vi "TDMS Record.vi"(9 "Data":dbl[][](array[numeric]), 10 "Input TDMS File Cluster":T1, 11 "In Use Cluster":T2) -> (3 "Output TDMS File Cluster":T1)   [LabVIEW 2014]
panel:
  # "TDMS Record VI"
  # "Inputs"
  # "Outputs"
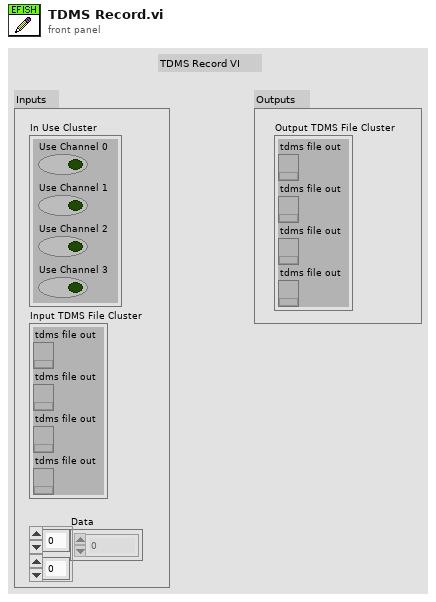
[diagram p1: front panel]
types:
  T1 = cluster{"tdms file out":refnum<k34>, "tdms file out":refnum<k34>, "tdms file out":refnum<k34>, "tdms file out":refnum<k34>}
  T2 = cluster{"Use Channel 0":bool, "Use Channel 1":bool, "Use Channel 2":bool, "Use Channel 3":bool}
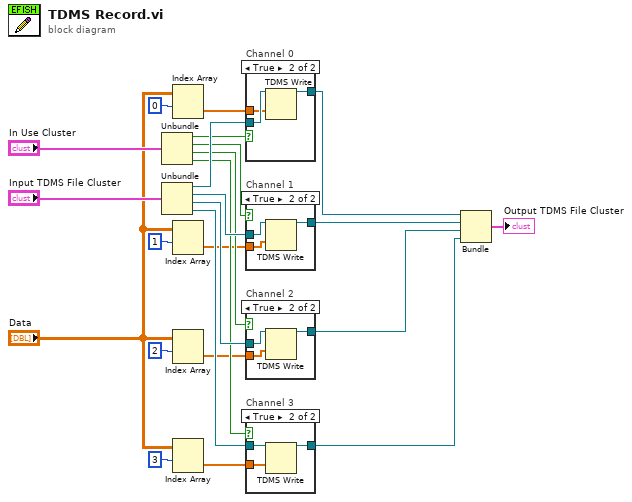
[diagram p0: block diagram]
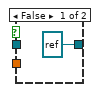
[diagram p2: hidden frame]
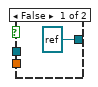
[diagram p3: hidden frame]
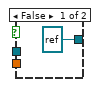
[diagram p4: hidden frame]
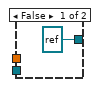
[diagram p5: hidden frame]
diagram:
  n1 = Unbundle("In Use Cluster") -> ("Use Channel 0"=w22:bool, "Use Channel 1"=w17:bool, "Use Channel 2"=w16:bool, "Use Channel 3"=w15:bool)
  n2 = Unbundle("Input TDMS File Cluster") -> ("tdms file out"=w24:refnum<k34>, "tdms file out"=w20:refnum<k34>, "tdms file out"=w19:refnum<k34>, "tdms file out"=w18:refnum<k34>)
  n3 = Index Array(array="Data", index (row)=0) -> (element=w13:dbl[])  [unwired: 1 in]
  n4 = Index Array(array="Data", index (row)=1) -> (element=w11:dbl[])  [unwired: 1 in]
  n5 = Index Array(array="Data", index (row)=2) -> (element=w9:dbl[])  [unwired: 1 in]
  n6 = Index Array(array="Data", index (row)=3) -> (element=w6:dbl[])  [unwired: 1 in]
  n7 = case "Channel 0" shown="True" w22 {
    tunnel: w24 -> [_ w28]
    tunnel: [refnum<k34> refnum ("tdms file out") w27] -> w5
    tunnel: w13 -> [_ w26]
    frame False {
    }
    frame True {
      n8 = TDMS Write(0:w28, 9:w26) -> (4:w27:refnum<k34>)  [unwired: 4 in, 3 out]
    }
  }
  n9 = case "Channel 1" shown="True" w17 {
    tunnel: [refnum<k34> refnum ("tdms file out") w32] -> w4
    tunnel: w20 -> [_ w31]
    tunnel: w11 -> [_ w30]
    frame False {
    }
    frame True {
      n10 = TDMS Write(0:w31, 9:w30) -> (4:w32:refnum<k34>)  [unwired: 4 in, 3 out]
    }
  }
  n11 = case "Channel 2" shown="True" w16 {
    tunnel: [refnum<k34> refnum ("tdms file out") w36] -> w3
    tunnel: w19 -> [_ w35]
    tunnel: w9 -> [_ w34]
    frame False {
    }
    frame True {
      n12 = TDMS Write(0:w35, 9:w34) -> (4:w36:refnum<k34>)  [unwired: 4 in, 3 out]
    }
  }
  n13 = case "Channel 3" shown="True" w15 {
    tunnel: [refnum<k34> refnum ("tdms file out") w40] -> w2
    tunnel: w18 -> [_ w39]
    tunnel: w6 -> [_ w38]
    frame False {
    }
    frame True {
      n14 = TDMS Write(0:w39, 9:w38) -> (4:w40:refnum<k34>)  [unwired: 4 in, 3 out]
    }
  }
  n15 = Bundle("tdms file out"=w5, "tdms file out"=w4, "tdms file out"=w3, "tdms file out"=w2) -> (→"Output TDMS File Cluster":T1)  [unwired: 1 in]
